vi "From String.vi"(6 "CConfig Encoding [Automatic]":refnum<class "CConfig Encoding.lvclass">=refnum, 8 "error in (no error)":errorcluster, 10 "String":string, 11 "Carya Config in":refnum<class "Carya Config.lvclass">) -> (0 "error out":errorcluster, 2 "Used encoding":refnum<class "CConfig Encoding.lvclass">, 3 "Carya Config out":refnum<class "Carya Config.lvclass">)   [LabVIEW 2013, in "Carya Config.lvclass"]
doc: "Copyright 2018, Carya Automatisering, Wiebe Walstra."
uses:
  Carya Config.lvclass
  CConfig Encoding/CConfig Encoding.lvclass
  CConfig Encoding/CConfig Automatic Encoding/CConfig Automatic Encoding.lvclass
  Carya Config.lvclass/Carya Config.ctl
  CConfig Object/CConfig Object.lvclass
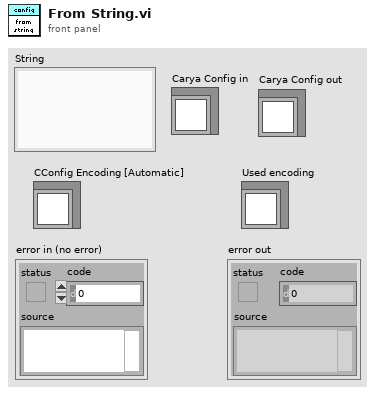
[diagram p1: front panel]
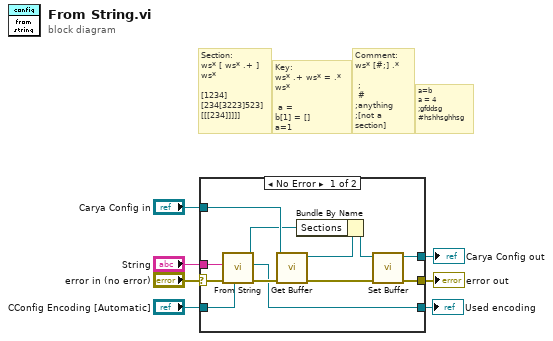
[diagram p0: block diagram]
diagram:
  # "Comment:\nws* [#;] .*\n\n ;\n #\n;anything\n;[not a section]"
  # "Key:\nws* .+ ws* = .* ws*\n\n a = \nb[1] = []\na=1"
  # "Section: \nws* [ ws* .+ ] ws*\n\n[1234]\n[234[3223]523]\n[[[234]]]]]"
  # "a=b\na = 4\n;gfddsg\n#hshhsghhsg"
  n1 = case shown="No Error" "error in (no error)" {
    selector: "error in (no error)" -> [w12 w21]
    tunnel: [w18 w21] -> w4
    tunnel: [w17 w20] -> w6
    tunnel: "Carya Config in" -> [w19 w20]
    tunnel: "String" -> [w14 _]
    tunnel: "CConfig Encoding [Automatic]" -> [w9 _]
    tunnel: [w8 _] -> w1
    frame No Error {
      n2 = call "From String.vi"("CConfig Encoding [Automatic]"=w9, "error in (no error)"=w12, "String"=w14) -> ("error out"=w11:errorcluster, "Used encoding"=w8:refnum<class "CConfig Encoding.lvclass">, "Section Object out"=w13:refnum<class "CConfig Object.lvclass">)  [unwired: 6 in]
      n3 = call-dynamic "Get Buffer.vi"("error in (no error)"=w11, "Carya Config in"=w19) -> ("error out"=w10:errorcluster, "Config"=w16:refnum<class "Carya Config.lvclass">)  [unwired: 8 in]
      n4 = Bundle By Name(cluster=w16, "Sections"=w13) -> (w15:refnum<class "Carya Config.lvclass">)
      n5 = call-dynamic "Set Buffer.vi"("error in (no error)"=w10, "Carya Config"=w15) -> ("error out"=w18:errorcluster, "Carya Config out"=w17:refnum<class "Carya Config.lvclass">)  [unwired: 8 in]
    }
    frame Error {
    }
  }
  "error out" <- w4
  "Carya Config out" <- w6
  "Used encoding" <- w1
